vi "NewRoomWithBomb.vi"(8 "error in (no error)":errorcluster, 10 "Bombed":bool, 11 "RoomNumber":i32) -> (0 "error out":errorcluster, 3 "RoomWithBomb":refnum<class "RoomWithBomb.lvclass">)   [LabVIEW 2020, in "RoomWithBomb.lvclass"]
uses:
  RoomWithBomb.lvclass
  RoomWithBomb.lvclass/RoomWithBomb.ctl
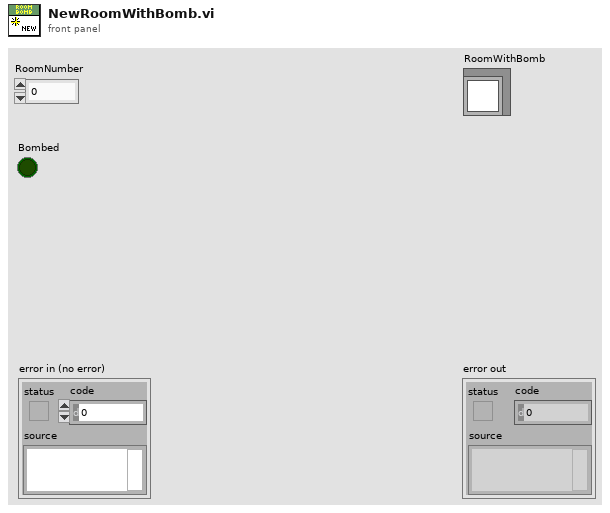
[diagram p1: front panel]
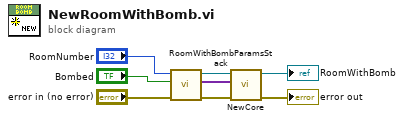
[diagram p0: block diagram]
diagram:
  n1 = call "RoomWithBombParamsStack.vi"("error in (no error)"="error in (no error)", "Bomb"="Bombed", "RoomNumber"="RoomNumber") -> ("error out"=w8:errorcluster, "HierarchyParams"=w7:variant[], "RoomWithBomb"=w6:refnum<class "RoomWithBomb.lvclass">)  [unwired: 6 in]
  n2 = call-dynamic "NewCore.vi"("error in (no error)"=w8, "ParamsArray"=w7, "RoomWithBomb"=w6) -> ("error out"=→"error out":errorcluster, "RoomWithBomb"=→"RoomWithBomb":refnum<class "RoomWithBomb.lvclass">)  [unwired: 7 in]
